vi "ep_Check U I Size Equal.vi"(8 "error in (no error)":errorcluster, 10 "current channel number":i32, 11 "voltage channel number":i32) -> (0 "error out":errorcluster)   [LabVIEW 2014, in "NI_EP_Motor Monitoring.lvlib"]
uses:
  <vilib>/addons/Electrical Power/Motor Monitoring/NI_EP_Motor Monitoring.lvlib
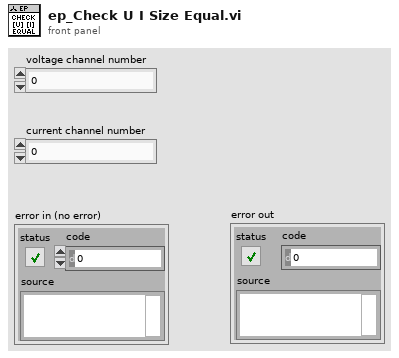
[diagram p1: front panel]
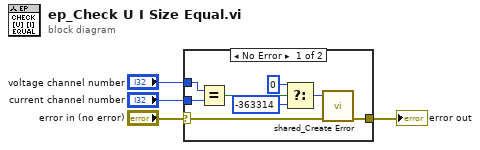
[diagram p0: block diagram]
diagram:
  n1 = case shown="No Error" "error in (no error)" {
    selector: "error in (no error)" -> [w7 w13]
    tunnel: [w6 w13] -> w3
    tunnel: "current channel number" -> [w12 _]
    tunnel: "voltage channel number" -> [w11 _]
    frame No Error {
      n2 = Equal?(x=w11, y=w12) -> (x = y?=w8:bool)
      n3 = Select(t=0, s=w8, f=-363314 ("error code (0)")) -> (s? t:f=w5:i32)
      n4 = call <vilib>:"shared_Create Error.vi"("error in (no error)"=w7, "error code (0)"=w5) -> ("error out"=w6:errorcluster)  [unwired: 9 in]
    }
    frame Error {
    }
  }
  "error out" <- w3
